vi "Get VI Ref from Name.vi"(8 "error in (no error)":errorcluster, 10 "VI Name":string, 11 "Model in":refnum<class "Model.lvclass">) -> (0 "error out":errorcluster, 1 "Found?":bool, 2 "VI Refnum":refnum<vi>, 3 "Model out":refnum<class "Model.lvclass">, 4 "Index":i32)   [LabVIEW 2015, in "Model.lvlib" / "Model.lvclass"]
uses:
  Model.lvclass
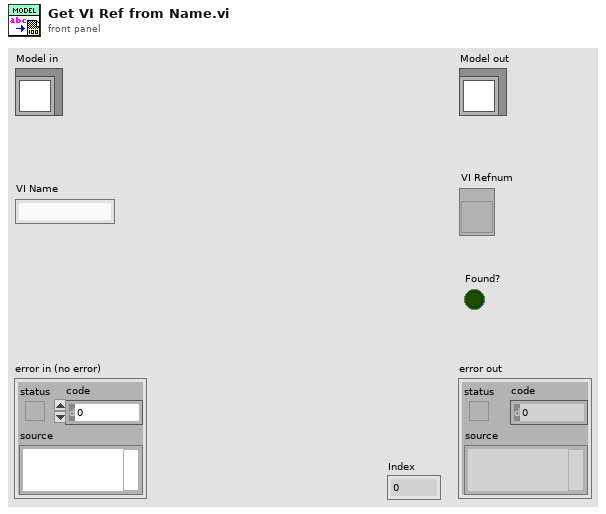
[diagram p1: front panel]
types:
  T1 = typedef "Model.lvlib/VI Infomation.ctl" = cluster{"Name":string, "Description":string, "Icon":picture}
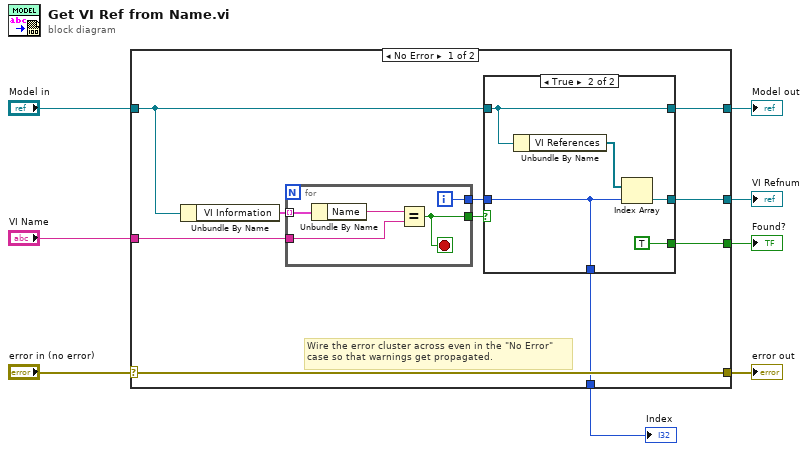
[diagram p0: block diagram]
diagram:
  n1 = case shown="No Error" "error in (no error)" {
    selector: "error in (no error)" -> [w18 w31]
    tunnel: [w18 w31] -> w7
    tunnel: [w12 w30] -> w5
    tunnel: "Model in" -> [w13 w30]
    tunnel: "VI Name" -> [w16 _]
    tunnel: [w11 _] -> w3
    tunnel: [w10 _] -> w2
    tunnel: [w9 _] -> w1
    frame No Error {
      # "Wire the error cluster across even in the \"No Error\"\ncase so that warnings get propagated."
      n2 = Unbundle By Name(w13) -> ("VI Information"=w17:T1[])
      n3 = for {
        tunnel: w17 -> [w29] mode=indexing
        tunnel: w16 -> [w27]
        tunnel: [w26] -> w15
        tunnel: [w25] -> w14
        i -> [w25]
        stop <- w26 stop-if-true
        n4 = Unbundle By Name(w29) -> ("Name"=w28:string)
        n5 = Equal?(x=w28, y=w27) -> (x = y?=w26:bool)
      }
      n6 = case shown="True" w15 {
        tunnel: w14 -> [_ w20]
        tunnel: w13 -> [w19 w23]
        tunnel: [w19 w23] -> w12
        tunnel: [_ w22] -> w11
        tunnel: [_ TRUE] -> w10
        tunnel: [_ w20] -> w9
        frame False {
        }
        frame True {
          n7 = Unbundle By Name(w23) -> ("VI References"=w24:refnum<vi>[])
          n8 = Index Array(array=w24, index=w20) -> (element=w22:refnum<vi>)
        }
      }
    }
    frame Error {
    }
  }
  "error out" <- w7
  "Model out" <- w5
  "VI Refnum" <- w3
  "Found?" <- w2
  "Index" <- w1
